vi "IterateTabControl.vi"(0 "Ctl Refnum in":refnum<vi>, 5 "ControlDoBase in":refnum<class "ControlActionBase.lvclass">, 7 "Control Path":string[](array[string]), 11 "error in (no error)":errorcluster) -> (4 "Ctl Refnum out":refnum<vi>, 6 "ControlDoBase out":refnum<class "ControlActionBase.lvclass">, 15 "error out":errorcluster)   [LabVIEW 2016, in "ControlActionBase.lvclass"]
uses:
  ControlActionBase.lvclass
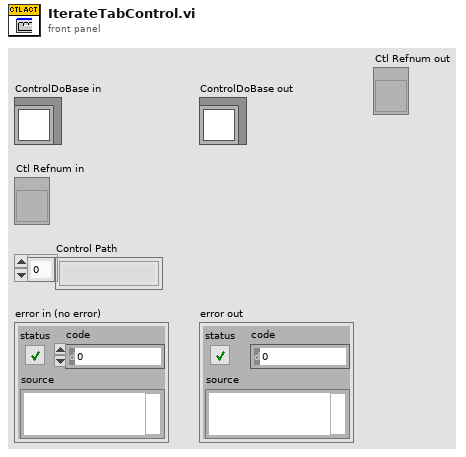
[diagram p1: front panel]
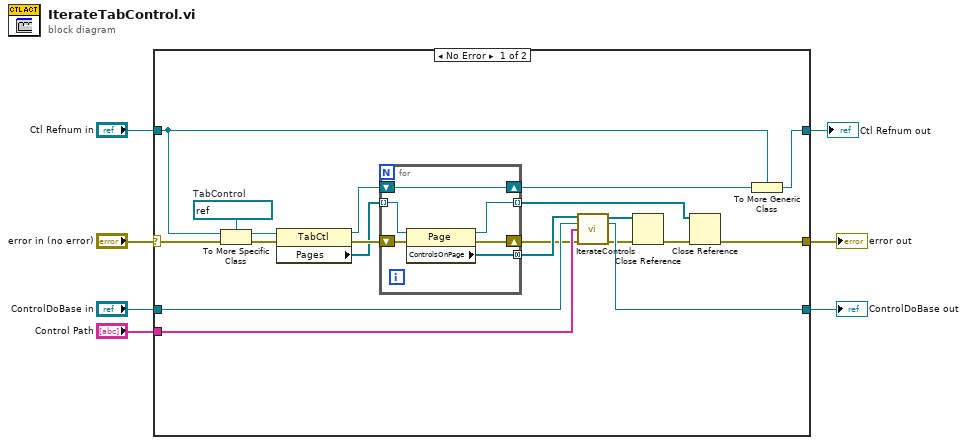
[diagram p0: block diagram]
diagram:
  n1 = case shown="No Error" "error in (no error)" {
    selector: "error in (no error)" -> [w24 w36]
    tunnel: [w27 w34] -> w7
    tunnel: [w26 w36] -> w6
    tunnel: "ControlDoBase in" -> [w23 w34]
    tunnel: "Control Path" -> [w22 _]
    tunnel: "Ctl Refnum in" -> [w9 w35]
    tunnel: [w8 w35] -> w1
    frame No Error {
      w13 = refnum<vi> refnum  # TabControl
      n2 = To More Specific Class(target class=w13, reference=w9, error in=w24) -> (specific class reference=w14:refnum<vi>, error out=w15:errorcluster)
      n3 = property class="TabCtl"(reference=w14, error in=w15) -> (reference out=w18:refnum<vi>, error out=w17:errorcluster, "Pages"=w16:refnum<vi>[])
      n4 = for {
        tunnel: w16 -> [w33] mode=indexing
        tunnel: [w32] -> w21 mode=concatenating
        shift-right: [w30] -> w19
        shift-left: w17 -> [w31]
        tunnel: [w29] -> w20 mode=indexing
        shift-right: [w28] -> w25
        shift-left: w18 -> [w28]
        n5 = property class="Page"(reference=w33, error in=w31) -> (reference out=w29:refnum<vi>, error out=w30:errorcluster, "ControlsOnPage"=w32:refnum<vi>[])
      }
      n6 = call-dynamic "IterateControls.vi"("Controls[] In"=w21, "ControlDoBase in"=w23, "Control Path"=w22, "error in (no error)"=w19) -> ("Controls[] Out"=w12:refnum<vi>[], "ControlDoBase out"=w27:refnum<class "ControlActionBase.lvclass">, "error out"=w10:errorcluster)  [unwired: 9 in]
      n7 = Close Reference(reference=w12, error in (no error)=w10) -> (error out=w11:errorcluster)
      n8 = Close Reference(reference=w20, error in (no error)=w11) -> (error out=w26:errorcluster)
      n9 = To More Generic Class(target class=w9, reference=w25) -> (generic class reference=w8:refnum<vi>)
    }
    frame Error {
    }
  }
  "ControlDoBase out" <- w7
  "error out" <- w6
  "Ctl Refnum out" <- w1
